vi "SVFA Map Order to Frequency.vi"(10 "speed [RPM]":dbl=3600.0 min=0.0 step=1.0, 11 "order":dbl=1.0 min=0.0 step=0.1) -> (3 "frequency [Hz]":dbl=nan)   [LabVIEW 2017]
doc: "Use this VI to convert an order power spectrum to a frequency power spectrum. Use this VI to convert power spectrum results from constant-speed applications."
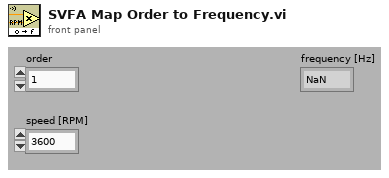
[diagram p1: front panel]
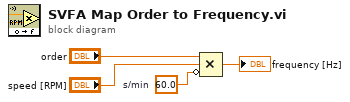
[diagram p0: block diagram]
diagram:
  w2 = 60.0  # s/min
  n1 = Compound Arithmetic op=MULTIPLY("order", "speed [RPM]", invert w2) -> (→"frequency [Hz]":dbl)
